vi "show_available_isotopes.vi"(8 "error in (no error)":errorcluster, 9 "Dataset":string(combo), 10 "Analysis in":refnum<class "Analysis.lvclass">, 11 "menu reference":refnum<k9>) -> (0 "error out":errorcluster)   [LabVIEW 2015]
doc: "looks into the selected dataset (extrapolatin results, scan data, SystemDevices) and finds the available isotopes/SysDevices.Those isotope names (or SystemDevice names) are added to the runtime menu under \"Plot\""
uses:
  MSControl/Classes/Analysis/Analysis.lvclass
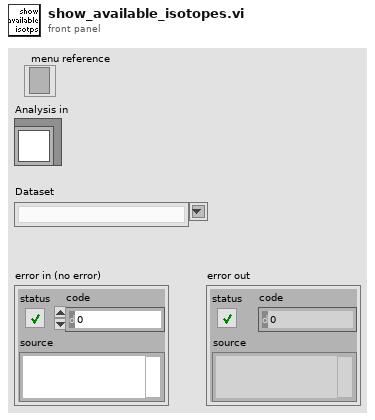
[diagram p1: front panel]
types:
  T1 = typedef "ExtrapolationResultsArray.ctl" = string[][]
  T2 = typedef "ScanDataArray_new.ctl" = cluster{"scan data":string[][]}[]
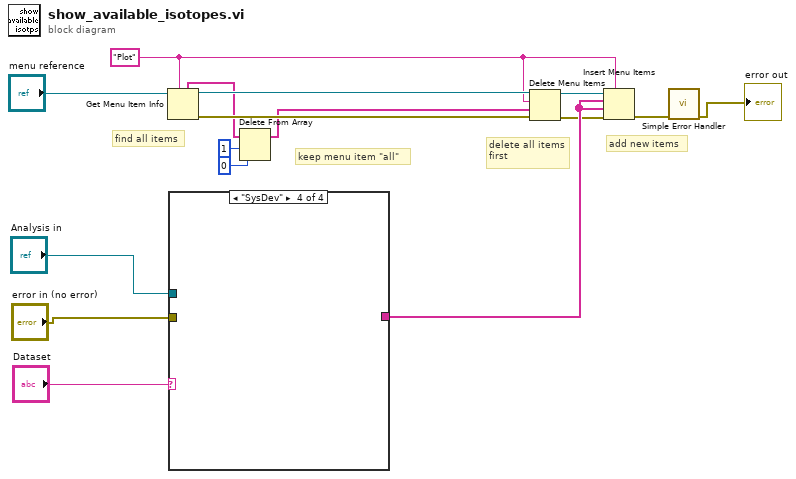
[diagram p0: block diagram]
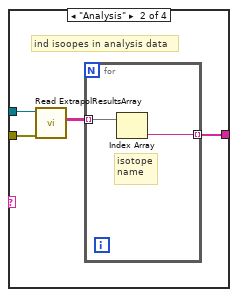
[diagram p3: hidden frame]
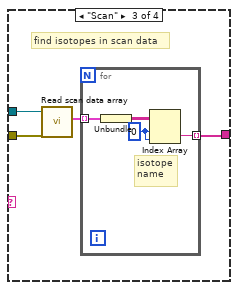
[diagram p4: hidden frame]
diagram:
  w5 = "Plot" ("menu tag")
  # "keep menu item \"all\""
  # "find all items"
  # "add new items"
  # "delete all items\nfirst"
  n1 = Get Menu Item Info(7:w5, 11:"menu reference") -> (0:w8:errorcluster, 3:w7:refnum<k9>, 5:w4:string[])  [unwired: 1 in, 4 out]
  n2 = case shown="\"SysDev\"" "Dataset" {
    tunnel: "Analysis in" -> [_ w19 w26 _]
    tunnel: "error in (no error)" -> [_ w18 w25 _]
    tunnel: [_ w17 w23 _] -> w14
    frame "False", Default {
    }
    frame "Analysis" {
      # "ind isoopes in analysis data"
      n3 = call-dynamic "Read ExtrapolResultsArray.vi"("error in (no error)"=w18, "Analysis in"=w19) -> ("ExtrapolResultsArray"=w20:T1)  [unwired: 7 in, 2 out]
      n4 = for {
        tunnel: w20 -> [w22] mode=indexing
        tunnel: [w21] -> w17 mode=indexing
        # "isotope\nname"
        n5 = Index Array(array=w22) -> (element=w21:string)  [unwired: 1 in]
      }
    }
    frame "Scan" {
      # "find isotopes in scan data"
      n6 = call-dynamic "Read scan data array.vi"("error in (no error)"=w25, "Analysis in"=w26) -> ("scan data array"=w24:T2)  [unwired: 7 in, 2 out]
      n7 = for {
        tunnel: w24 -> [w30] mode=indexing
        tunnel: [w27] -> w23 mode=indexing
        w28 = 0 ("index (row)")
        # "isotope\nname"
        n8 = Unbundle(w30) -> ("scan data"=w29:string[][])
        n9 = Index Array(array=w29, index (row)=w28, index (col)=w28) -> (element=w27:string)
      }
    }
    frame "SysDev" {
    }
  }
  n10 = Delete From Array(array=w4, length=1, index=0) -> (array with subset deleted=w1:string[])  [unwired: 1 out]
  n11 = Delete Menu Items(6:w8, 7:w1, 8:w5, 9:w7) -> (0:w9:errorcluster, 3:w10:refnum<k9>)
  n12 = Insert Menu Items(5:w5, 6:w9, 7:w14, 8:w14, 9:w10) -> (0:w13:errorcluster)  [unwired: 1 in, 2 out]
  n13 = call <vilib>:"Simple Error Handler.vi"("error in (no error)"=w13) -> ("error out"=→"error out":errorcluster)  [unwired: 4 in, 4 out]
